vi "Get-Ctrl-Ref's & Label's.vi"(0 "VI Refnum":refnum<vi>, 11 "error in (no error)":errorcluster) -> (4 "Quick-GUI-Update out":refnum<class "Quick-GUI-Update.lvclass">, 8 "Label's List":string[][](array[string]), 15 "error out":errorcluster)   [LabVIEW 2020, in "Quick-GUI-Update.lvclass"]
uses:
  Quick-GUI-Update.lvclass
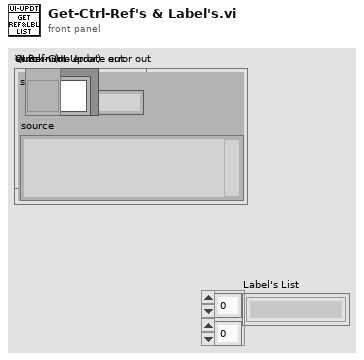
[diagram p1: front panel]
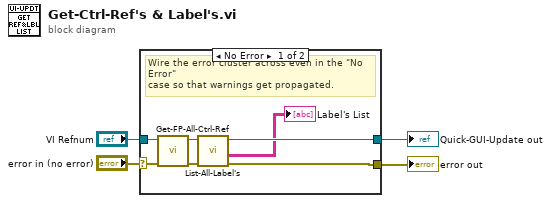
[diagram p0: block diagram]
diagram:
  n1 = case shown="No Error" "error in (no error)" {
    selector: "error in (no error)" -> [w6 w12]
    tunnel: [w10 w12] -> w3
    tunnel: [w11 _] -> w2
    tunnel: "VI Refnum" -> [w5 _]
    frame No Error {
      # "Wire the error cluster across even in the \"No Error\"\ncase so that warnings get propagated."
      n2 = call "Get-FP-All-Ctrl-Ref.vi"("error in (no error)"=w6, "VI Refnum"=w5) -> ("error out"=w8:errorcluster, "Quick-GUI-Update out"=w7:refnum<class "Quick-GUI-Update.lvclass">)  [unwired: 8 in]
      n3 = call "List-All-Label's.vi"("error in (no error)"=w8, "Quick-GUI-Update in"=w7) -> ("error out"=w10:errorcluster, "Label's List"=→"Label's List":string[][], "Quick-GUI-Update out"=w11:refnum<class "Quick-GUI-Update.lvclass">)  [unwired: 7 in]
    }
    frame Error {
    }
  }
  "error out" <- w3
  "Quick-GUI-Update out" <- w2
